vi "Модель.vi"() -> ()   [LabVIEW 2013]
uses:
  <vilib>/Analysis/2dsp.llb/Real FFT.vi
  <vilib>/Analysis/2dsp.llb/Inverse Real FFT.vi
  <vilib>/addons/Modulation/Digital/Channel Coding/MT Hamming Encoder (Systematic).vi
  <vilib>/addons/Modulation/Analog/MT Modulate AM (DSB).vi
  <vilib>/addons/Modulation/Analog/MT Upconvert Baseband (Real).vi
  <vilib>/measure/maspectr.llb/FFT Power Spectrum and PSD for 1 Chan.vi
  <vilib>/Utility/file.llb/Read From Spreadsheet File (DBL).vi
  <vilib>/addons/Modulation/niAMT.lvlib
  <vilib>/addons/Modulation/niDMT.lvlib
  <vilib>/Analysis/NI_AALPro.lvlib
  <vilib>/measure/NI_MAPro.lvlib
panel:
  out "size(s) 2":i32
  in  "Tab Control":T1(tab)
  out "Waveform Graph 2":dbl[](graph)
  out "Waveform Graph":dbl[](graph)
  out "Tx Signal Spectrum":cluster{"f0":dbl, "df":dbl, "magnitude":dbl[]}(graph)
  out "Tx Signal":waveform(dbl)(graph)
  out "Rx Signal":waveform(dbl)(graph)
  in  "Spreadsheet path (.csv) 2":path=path "C:/Users/husmith/Desktop/MyData.csv"
  out "output array":dbl[](array[numeric])
  out "size(s)":i32
  in  "carrier frequency (Hz)":dbl=8000000000.0 min=-0.5 max=0.5 format="%.2f"
  in  "PPM Input Level":u8(slide)=50 step=1 scale=50.0..310.0
  in  "Modulation Index":dbl=0.8 min=0.0 step=0.01 format="%#.3f"
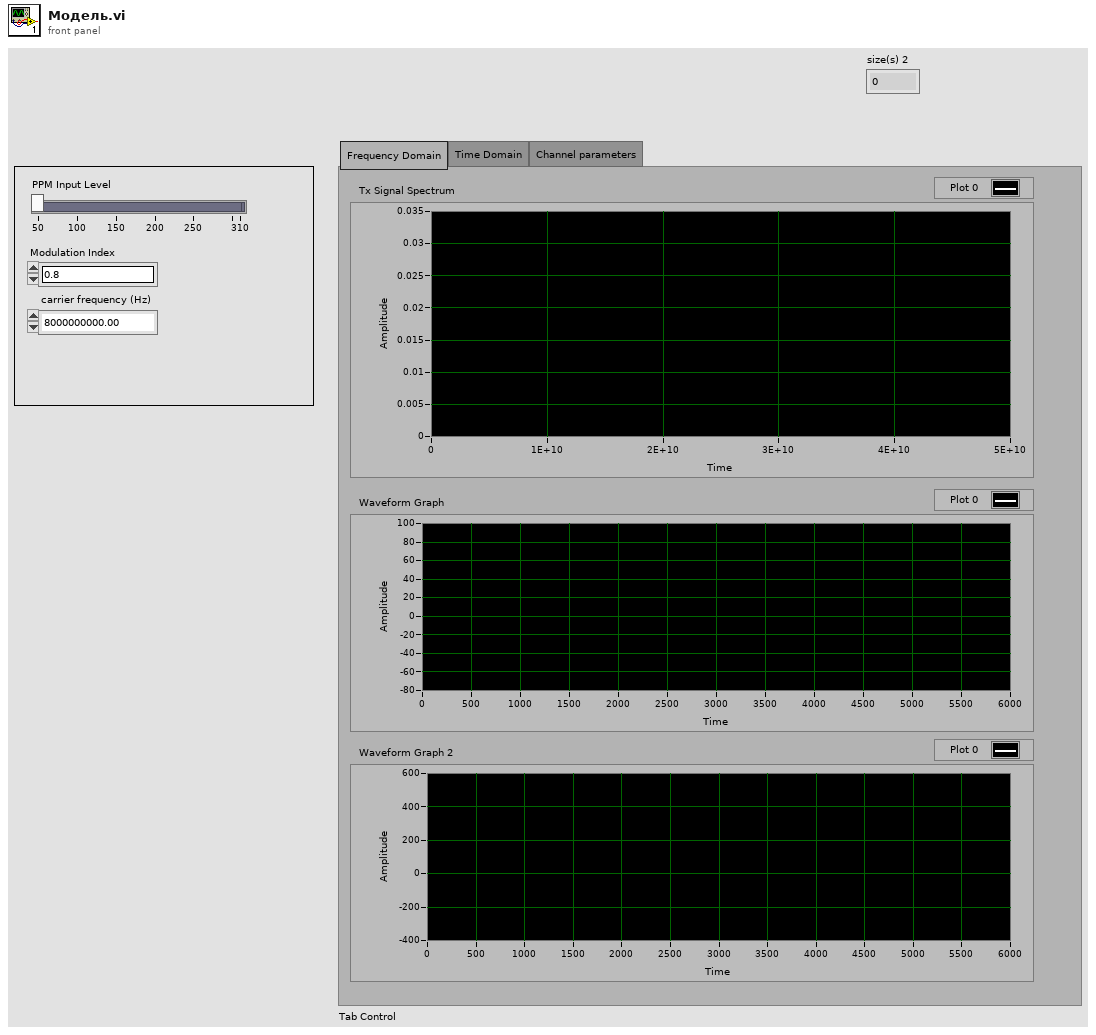
[diagram p1: front panel]
types:
  T1 = enum32{"Frequency Domain", "Time Domain", "Channel parameters"}
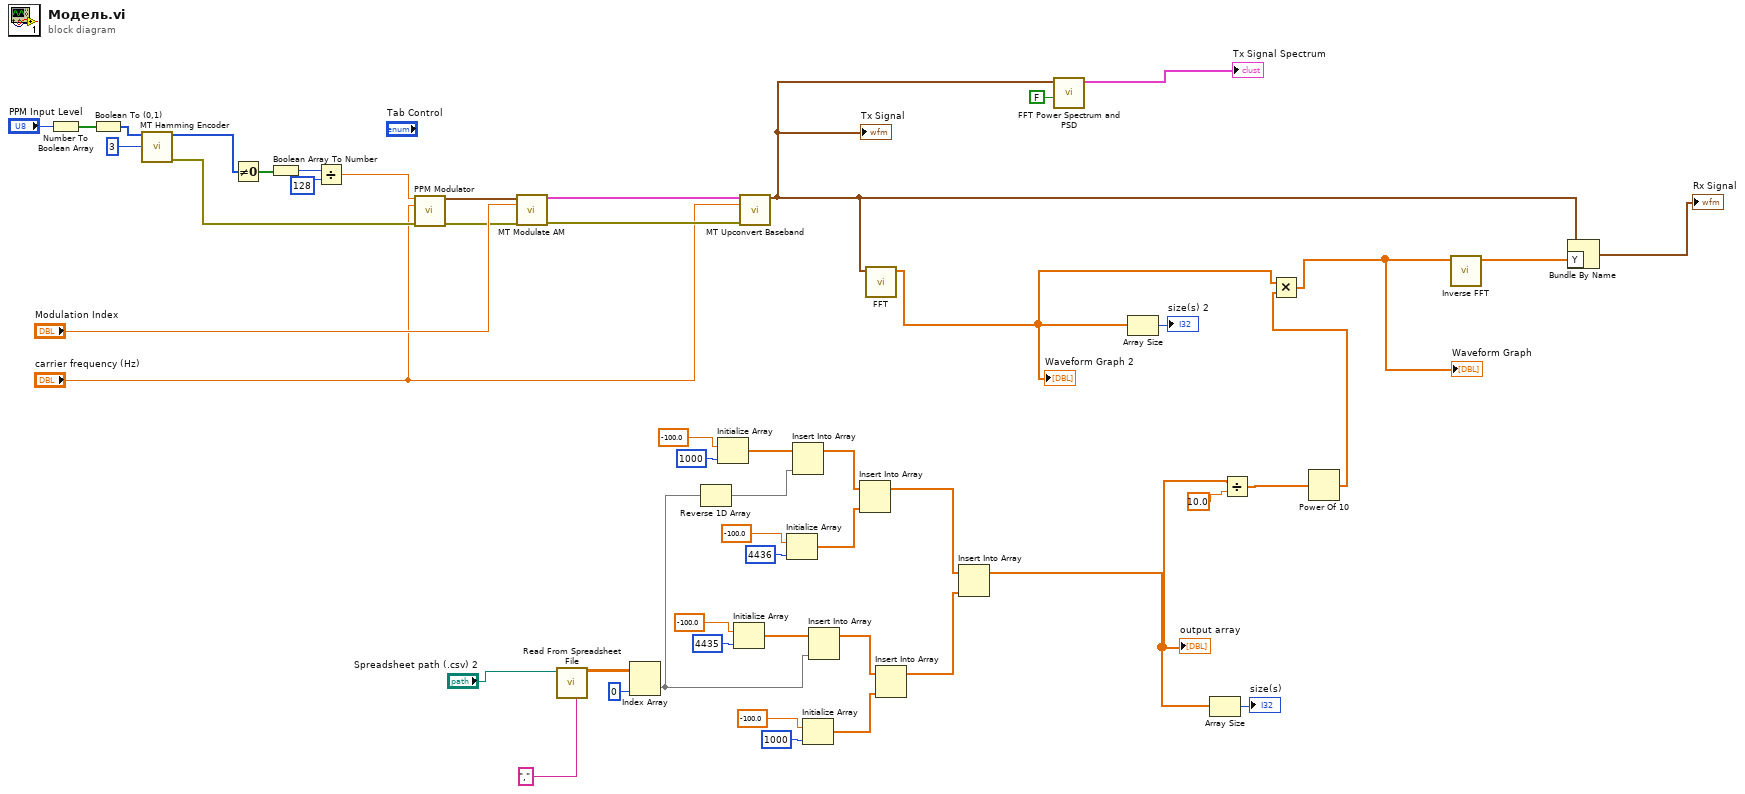
[diagram p0: block diagram]
diagram:
  n1 = Number To Boolean Array(number="PPM Input Level") -> (Boolean array=w47:bool[])
  n2 = Boolean To (0,1)(Boolean=w47) -> (0, 1=w44:i16[])
  n3 = call-poly <vilib>:"MT Hamming Encoder.vi"("input bit stream"=w44, "hamming order"=3) -> ("output bit stream"=w45:i8[], "error out"=w37:errorcluster)  [unwired: 12 in]
  n4 = Not Equal To 0?(x=w45) -> (x != 0?=w46:bool[])
  n5 = Boolean Array To Number(Boolean array=w46) -> (number=w43:u32)
  n6 = Divide(x=w43, y=u32 128) -> (x/y=w41:dbl)
  n7 = call "PPM Modulator.vi"("Input level"=w41, "Carrier Frequency(Hz)"="carrier frequency (Hz)", "error in (no error)"=w37) -> ("PPM with Sync"=w51:waveform(dbl), "error out"=w38:errorcluster)  [unwired: 10 in, 1 out]
  n8 = call-poly <vilib>:"MT Modulate AM.vi"("message signal"=w51, "modulation index"="Modulation Index", "error in (no error)"=w38) -> ("AM modulated waveform"=w40:cluster{"t0":dbl, "dt":dbl, "Y":cdb[]}, "error out"=w39:errorcluster)  [unwired: 11 in]
  n9 = call-poly <vilib>:"Read From Spreadsheet File.vi"("delimiter (\\t)"="," ("delimiter (\\t)"), "file path (dialog if empty)"="Spreadsheet path (.csv) 2") -> ("all rows"=w26:dbl[][])  [unwired: 5 in, 4 out]
  n10 = Index Array(array=w26, index (col)=0 ("index (row)")) -> (element=w7:dbl[])  [unwired: 1 in]
  n11 = Reverse 1D Array(array=w7) -> (reversed array=w8:dbl[])
  n12 = Initialize Array(-100.0 ("element"), 1000 ("dimension size")) -> (w11:dbl[])
  n13 = Initialize Array(-100.0 ("element"), 4435 ("dimension size")) -> (w27:dbl[])
  n14 = call-poly <vilib>:"MT Upconvert Baseband.vi"("baseband waveform (complex)"=w40, "carrier frequency (Hz)"="carrier frequency (Hz)", "error in (no error)"=w39) -> ("passband waveform"=w21:waveform(dbl))  [unwired: 11 in, 1 out]
  "Tx Signal" <- w21
  n15 = Initialize Array(-100.0 ("element"), 4436 ("dimension size")) -> (w9:dbl[])
  n16 = Insert Into Array(array=w11, new element=w8) -> (w10:dbl[])  [unwired: 1 in]
  n17 = Initialize Array(-100.0 ("element"), 1000 ("dimension size")) -> (w23:dbl[])
  n18 = Insert Into Array(array=w27, new element=w7) -> (w24:dbl[])  [unwired: 1 in]
  n19 = Insert Into Array(array=w10, new element=w9) -> (w6:dbl[])  [unwired: 1 in]
  n20 = call-poly <vilib>:"FFT.vi"("X"=w21) -> ("FFT {X}"=w1:cdb[])  [unwired: 9 in, 1 out]
  "Waveform Graph 2" <- w1
  n21 = Insert Into Array(array=w24, new element=w23) -> (w5:dbl[])  [unwired: 1 in]
  n22 = Insert Into Array(array=w6, new element=w5) -> (w4:dbl[])  [unwired: 1 in]
  "output array" <- w4
  n23 = call-poly <vilib>:"FFT Power Spectrum and PSD.vi"("dB On (F)"=FALSE, "time signal"=w21) -> ("Power Spectrum / PSD"=→"Tx Signal Spectrum":cluster{"f0":dbl, "df":dbl, "magnitude":dbl[]})  [unwired: 6 in, 3 out]
  n24 = Array Size(array=w1) -> (size(s)=→"size(s) 2":i32)
  n25 = Array Size(array=w4) -> (size(s)=→"size(s)":i32)
  n26 = Divide(x=w4, y=10.0) -> (x/y=w18:dbl[])
  n27 = Power Of 10(x=w18) -> (10^x=w3:dbl[])
  n28 = Multiply(x=w1, y=w3) -> (x*y=w2:cdb[])
  "Waveform Graph" <- w2
  n29 = call-poly <vilib>:"Inverse FFT.vi"("FFT {X}"=w2) -> ("X"=w16:dbl[])  [unwired: 9 in, 1 out]
  n30 = Bundle By Name(cluster=w21, "Y"=w16) -> (→"Rx Signal":waveform(dbl))
